vi "SSC_Compute_Legacy.vi"(9 "Tube Length":dbl format="%.6f", 10 "Cal Tube Temp":dbl, 11 "Sound Tube Temp":dbl[](array[numeric])) -> (3 "SSC Out(m)":dbl)   [LabVIEW 2019]
uses:
  <vilib>/Analysis/baseanly.llb/Mean (DBL).vi
  <vilib>/Analysis/NI_AALBase.lvlib
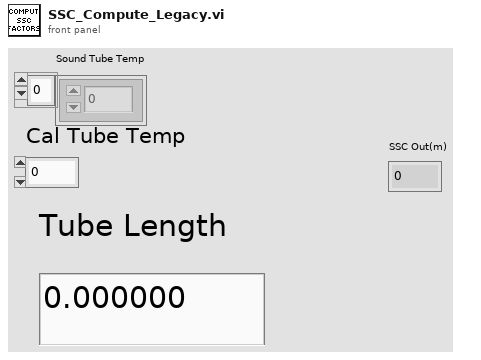
[diagram p1: front panel]
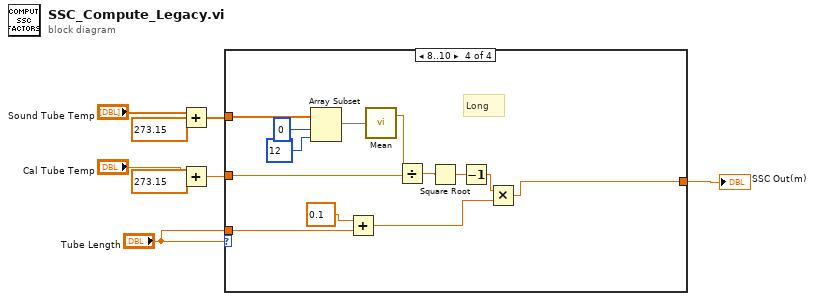
[diagram p0: block diagram]
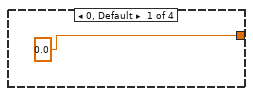
[diagram p2: hidden frame]
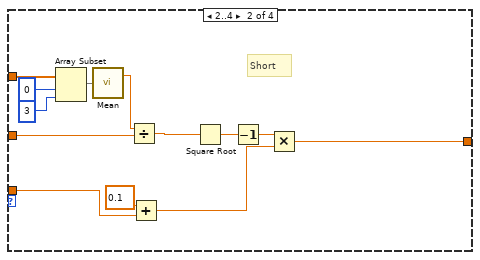
[diagram p3: hidden frame]
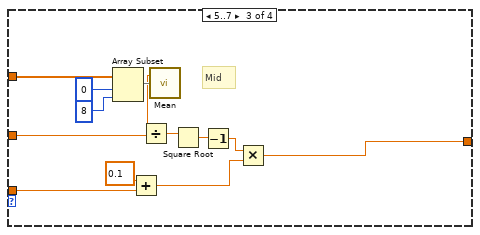
[diagram p4: hidden frame]
diagram:
  n1 = Add(x="Sound Tube Temp", y=273.15) -> (x+y=w3:dbl[])
  n2 = Add(x="Cal Tube Temp", y=273.15) -> (x+y=w5:dbl)
  n3 = case shown="8..10" "Tube Length" {
    tunnel: w3 -> [_ w22 w35 w48]
    tunnel: "Tube Length" -> [_ w18 w31 w44]
    tunnel: w5 -> [_ w14 w27 w40]
    tunnel: [0.0 w10 w23 w36] -> w1
    frame 0, Default {
    }
    frame 2..4 {
      # "Short"
      n4 = Array Subset(array=w22, index=0, length=3) -> (w16:dbl[])
      n5 = call-poly <vilib>:"Mean.vi"("X"=w16) -> ("mean"=w15:dbl)  [unwired: 1 out]
      n6 = Divide(x=w15, y=w14) -> (x/y=w13:dbl)
      n7 = Add(x=0.1 ("y"), y=w18) -> (x+y=w19:dbl)
      n8 = Square Root(x=w13) -> (sqrt(x)=w12:dbl)
      n9 = Decrement(x=w12) -> (x-1=w11:dbl)
      n10 = Multiply(x=w11, y=w19) -> (x*y=w10:dbl)
    }
    frame 5..7 {
      # "Mid"
      n11 = Array Subset(array=w35, index=0, length=8) -> (w29:dbl[])
      n12 = Add(x=0.1 ("y"), y=w31) -> (x+y=w32:dbl)
      n13 = call-poly <vilib>:"Mean.vi"("X"=w29) -> ("mean"=w28:dbl)  [unwired: 1 out]
      n14 = Divide(x=w28, y=w27) -> (x/y=w26:dbl)
      n15 = Square Root(x=w26) -> (sqrt(x)=w25:dbl)
      n16 = Decrement(x=w25) -> (x-1=w24:dbl)
      n17 = Multiply(x=w24, y=w32) -> (x*y=w23:dbl)
    }
    frame 8..10 {
      # "Long"
      n18 = Array Subset(array=w48, index=0, length=12) -> (w42:dbl[])
      n19 = Add(x=0.1 ("y"), y=w44) -> (x+y=w45:dbl)
      n20 = call-poly <vilib>:"Mean.vi"("X"=w42) -> ("mean"=w41:dbl)  [unwired: 1 out]
      n21 = Divide(x=w41, y=w40) -> (x/y=w39:dbl)
      n22 = Square Root(x=w39) -> (sqrt(x)=w38:dbl)
      n23 = Decrement(x=w38) -> (x-1=w37:dbl)
      n24 = Multiply(x=w37, y=w45) -> (x*y=w36:dbl)
    }
  }
  "SSC Out(m)" <- w1
